vi "read flow and pid.vi"(6 "odor 2 setpoint":dbl, 7 "numPidReadings":i32=83, 8 "error in":errorcluster, 9 "odor 1 setpoint":dbl, 10 "air flow set point":dbl, 11 "daqmx tasks":T2) -> (0 "error out":errorcluster, 2 "flow rates":T1, 3 "pid reading":dbl format="%0.2f")   [LabVIEW 2013]
uses:
  <vilib>/DAQmx/read.llb/DAQmx Read (Analog DBL 1Chan 1Samp).vi
  <vilib>/DAQmx/read.llb/DAQmx Read (Analog 1D DBL 1Chan NSamp).vi
  <vilib>/Analysis/baseanly.llb/Mean (DBL).vi
  <vilib>/DAQmx/miscellaneous.llb/DAQmx Fill In Error Info.vi
  <vilib>/Analysis/NI_AALBase.lvlib
panel:
  in  "co2 setpoint":dbl
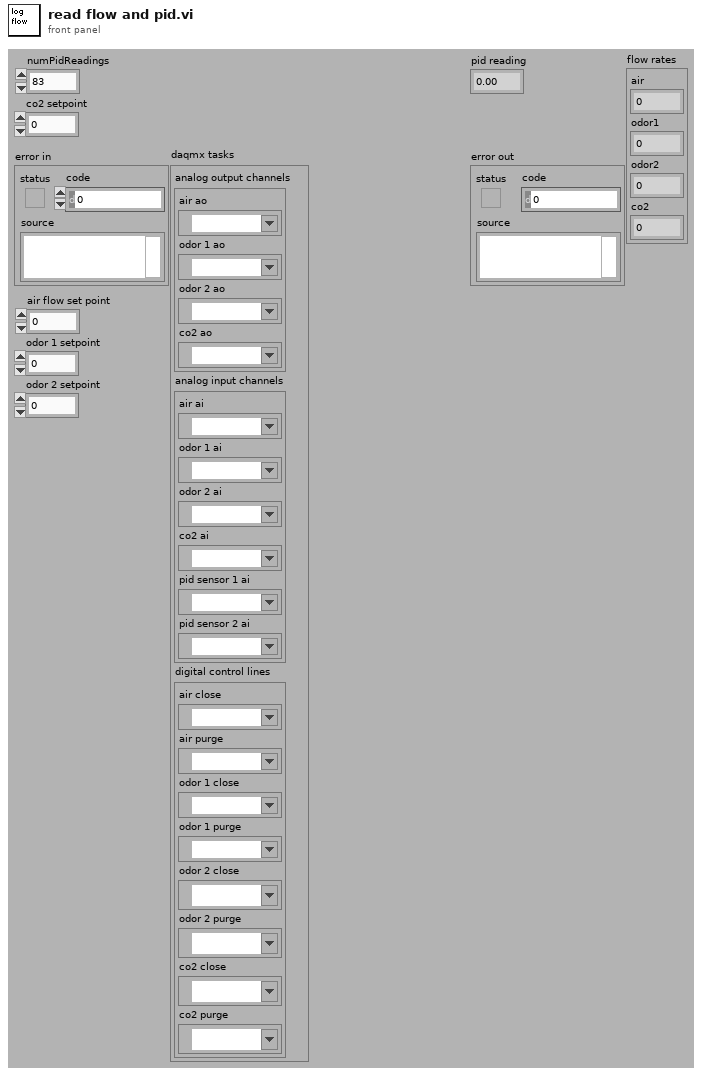
[diagram p1: front panel]
types:
  T1 = cluster{"air":dbl, "odor1":dbl, "odor2":dbl, "co2":dbl}
  T2 = cluster{"analog output channels":cluster{"air ao":refnum<k21>, "odor 1 ao":refnum<k21>, "odor 2 ao":refnum<k21>, "co2 ao":refnum<k21>}, "analog input channels":cluster{"air ai":refnum<k21>, "odor 1 ai":refnum<k21>, "odor 2 ai":refnum<k21>, "co2 ai":refnum<k21>, "pid sensor 1 ai":refnum<k21>, "pid sensor 2 ai":refnum<k21>}, "digital control lines":cluster{"air close":refnum<k21>, "air purge":refnum<k21>, "odor 1 close":refnum<k21>, "odor 1 purge":refnum<k21>, "odor 2 close":refnum<k21>, "odor 2 purge":refnum<k21>, "co2 close":refnum<k21>, "co2 purge":refnum<k21>}}
  T3 = enum16{"Reset Table", "Get Values", "Add Value", "Get Table", "Get Spreadsheet", "set stack writer"}
  T4 = cluster{"data":dbl, "data":dbl, "data":dbl, "data":dbl}
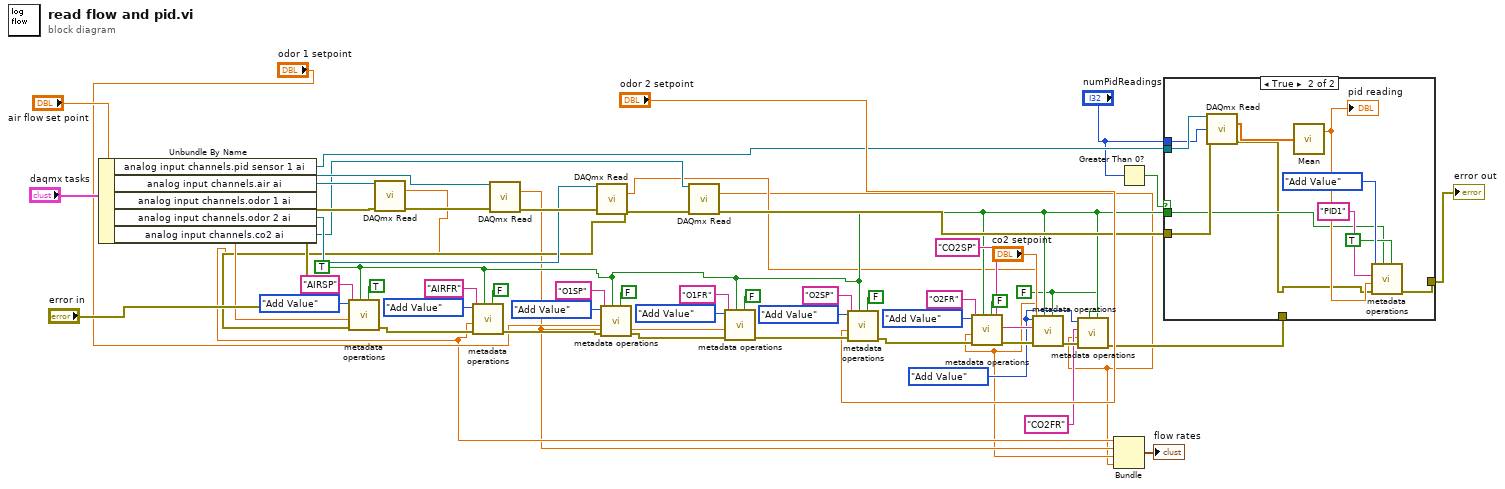
[diagram p0: block diagram]
diagram:
  w12 = T3."Add Value" ("Operation")
  w10 = FALSE ("add time?")
  w11 = TRUE ("add to stack writer")
  n1 = Unbundle By Name("daqmx tasks") -> ("analog input channels.pid sensor 1 ai"=w21:refnum<k21>, "analog input channels.air ai"=w52:refnum<k21>, "analog input channels.odor 1 ai"=w50:refnum<k21>, "analog input channels.odor 2 ai"=w48:refnum<k21>, "analog input channels.co2 ai"=w17:refnum<k21>)
  n2 = call-poly <vilib>:"DAQmx Read.vi"("task/channels in"=w52, "error in"="error in") -> ("data"=w5:dbl, "error out"=w51:errorcluster)  [unwired: 11 in, 1 out]
  n3 = call-poly <vilib>:"DAQmx Read.vi"("task/channels in"=w50, "error in"=w51) -> ("data"=w4:dbl, "error out"=w49:errorcluster)  [unwired: 11 in, 1 out]
  n4 = call-poly <vilib>:"DAQmx Read.vi"("task/channels in"=w48, "error in"=w49) -> ("data"=w3:dbl, "error out"=w19:errorcluster)  [unwired: 11 in, 1 out]
  n5 = call "metadata operations.vi"("add time?"=TRUE, "add to stack writer"=w11, "error in (no error)"=w19, "value"="air flow set point", "key"="AIRSP", "Operation"=T3."Add Value") -> ("error out"=w41:errorcluster)  [unwired: 2 in, 3 out]
  n6 = call "metadata operations.vi"("add time?"=FALSE, "add to stack writer"=w11, "error in (no error)"=w41, "value"=w5, "key"="AIRFR", "Operation"=T3."Add Value") -> ("error out"=w34:errorcluster)  [unwired: 2 in, 3 out]
  n7 = call "metadata operations.vi"("add time?"=FALSE, "add to stack writer"=w11, "error in (no error)"=w34, "value"="odor 1 setpoint", "key"="O1SP", "Operation"=T3."Add Value") -> ("error out"=w35:errorcluster)  [unwired: 2 in, 3 out]
  n8 = call-poly <vilib>:"DAQmx Read.vi"("task/channels in"=w17, "error in"=w19) -> ("data"=w2:dbl, "error out"=w18:errorcluster)  [unwired: 11 in, 1 out]
  n9 = call "metadata operations.vi"("add time?"=FALSE, "add to stack writer"=w11, "error in (no error)"=w35, "value"=w4, "key"="O1FR", "Operation"=T3."Add Value") -> ("error out"=w27:errorcluster)  [unwired: 2 in, 3 out]
  n10 = call "metadata operations.vi"("add time?"=FALSE, "add to stack writer"=w11, "error in (no error)"=w27, "value"="odor 2 setpoint", "key"="O2SP", "Operation"=T3."Add Value") -> ("error out"=w28:errorcluster)  [unwired: 2 in, 3 out]
  n11 = call "metadata operations.vi"("add time?"=FALSE, "add to stack writer"=w11, "error in (no error)"=w28, "value"=w3, "key"="O2FR", "Operation"=T3."Add Value") -> ("error out"=w16:errorcluster)  [unwired: 2 in, 3 out]
  n12 = call "metadata operations.vi"("add time?"=w10, "add to stack writer"=w11, "error in (no error)"=w16, "value"="co2 setpoint", "key"="CO2SP", "Operation"=w12) -> ("error out"=w13:errorcluster)  [unwired: 2 in, 3 out]
  n13 = call "metadata operations.vi"("add time?"=w10, "add to stack writer"=w11, "error in (no error)"=w13, "value"=w2, "key"="CO2FR", "Operation"=w12) -> ("error out"=w6:errorcluster)  [unwired: 2 in, 3 out]
  n14 = Bundle("data"=w5, "data"=w4, "data"=w3, "data"=w2) -> (→"flow rates":T4)  [unwired: 1 in]
  n15 = Greater Than 0?(x="numPidReadings") -> (x > 0?=w7:bool)
  n16 = case shown="True" w7 {
    tunnel: w21 -> [_ w66]
    tunnel: "numPidReadings" -> [_ w64]
    tunnel: [w55 w63] -> w20
    tunnel: w18 -> [_ w58]
    tunnel: w11 -> [_ w57]
    tunnel: w6 -> [w55 _]
    frame False {
    }
    frame True {
      n17 = call-poly <vilib>:"DAQmx Read.vi"("task/channels in"=w66, "number of samples per channel"=w64, "error in"=w58) -> ("data"=w65:dbl[], "error out"=w56:errorcluster)  [unwired: 10 in, 1 out]
      n18 = call-poly <vilib>:"Mean.vi"("X"=w65) -> ("mean"=w60:dbl)  [unwired: 1 out]
      "pid reading" <- w60
      n19 = call "metadata operations.vi"("add time?"=TRUE, "add to stack writer"=w57, "error in (no error)"=w56, "value"=w60, "key"="PID1", "Operation"=T3."Add Value") -> ("error out"=w63:errorcluster)  [unwired: 2 in, 3 out]
    }
  }
  "error out" <- w20
